vi "KDC101_Goto.vi"(5 "ErrRange(deg)":dbl=0.5, 6 "PositionRef":refnum<vi>, 7 "Position(deg)":dbl, 8 "error in (no error)":errorcluster caption="entrée d'erreur (pas d'erreur)", 9 "MovingRef":refnum<vi>, 10 "StopRef":refnum<vi>, 11 "KCubeDCServoRef":refnum<k24>) -> (0 "error out":errorcluster caption="sortie d'erreur", 1 "In Position":bool, 2 "PositionOut(deg)":dbl, 3 "KCubeDCServoRefOut":refnum<k24>)   [LabVIEW 2019]
doc: "Utilisez ce modèle pour construire un VI à utiliser en tant que sous-VI."
uses:
  C:/Program Files (x86)/National Instruments/LabVIEW 2019/user.lib/ThorKDC101/Kinesis_with_LabVIEW_Examples_LV12 - v3/ThorLabs.MotionControl.KCube.DCServoCLI.dll
  Kinesis_with_LabVIEW_Examples_LV12 - v3/ThorLabs.MotionControl.KCube.DCServoCLI.dll
  C:/Program Files (x86)/National Instruments/LabVIEW 2019/user.lib/ThorKDC101/Kinesis_with_LabVIEW_Examples_LV12 - v3/Thorlabs.MotionControl.GenericMotorCLI.dll
  Kinesis_with_LabVIEW_Examples_LV12 - v3/Thorlabs.MotionControl.GenericMotorCLI.dll
panel:
  in  "Stop":bool
  out "Moving":bool
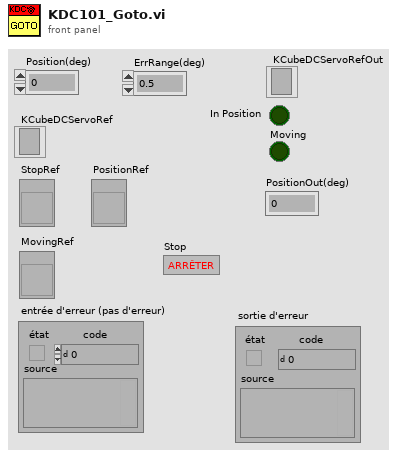
[diagram p1: front panel]
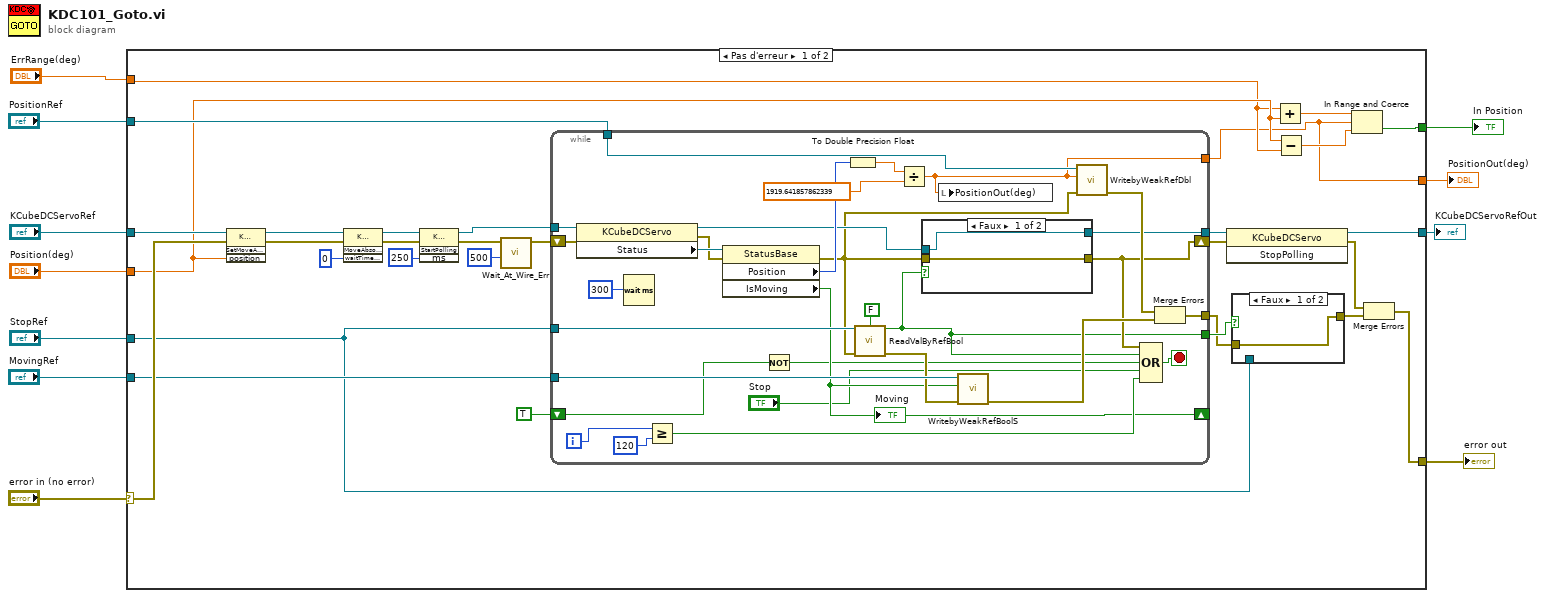
[diagram p0: block diagram]
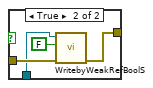
[diagram p2: hidden frame]
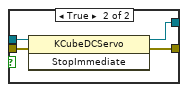
[diagram p3: hidden frame]
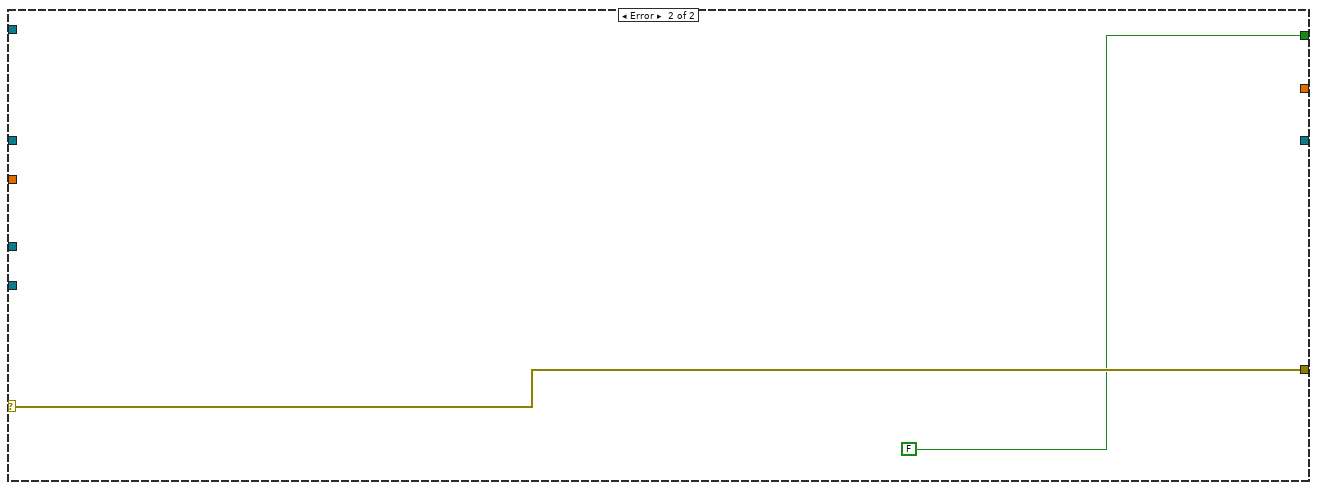
[diagram p4: hidden frame]
diagram:
  n1 = case shown="Pas d'erreur" "error in (no error)" {
    selector: "error in (no error)" -> [w37 w84]
    tunnel: [w33 w84] -> w10
    tunnel: [w17 FALSE] -> w9
    tunnel: "KCubeDCServoRef" -> [w40 _]
    tunnel: "MovingRef" -> [w34 _]
    tunnel: [w31 _] -> w6
    tunnel: "StopRef" -> [w13 _]
    tunnel: "Position(deg)" -> [w21 _]
    tunnel: "PositionRef" -> [w22 _]
    tunnel: "ErrRange(deg)" -> [w20 _]
    tunnel: [w16 _] -> w1
    frame No Error {
      n2 = invoke class="KCubeDCServo" method="SetMoveAbsolutePosition"(reference=w40, error in=w37, "position"=w21) -> (reference out=w27:refnum<k24>, error out=w28:errorcluster)  [unwired: 1 in, 2 out]
      n3 = invoke class="KCubeDCServo" method="MoveAbsolute"(reference=w27, error in=w28, "waitTimeout"=0) -> (reference out=w26:refnum<k24>, error out=w25:errorcluster)  [unwired: 1 in, 2 out]
      n4 = invoke class="KCubeDCServo" method="StartPolling"(reference=w26, error in=w25, "ms"=250) -> (reference out=w35:refnum<k24>, error out=w36:errorcluster)  [unwired: 1 in, 2 out]
      n5 = call <userlib>:"Wait_At_Wire_Err.vi"("Wait (ms)"=u32 500, "error in (no error)"=w36) -> ("error out"=w39:errorcluster)  [unwired: 7 in, 2 out]
      n6 = while {
        tunnel: [w54] -> w32
        tunnel: w35 -> [w75]
        tunnel: w34 -> [w70]
        shift-right: [w56] -> w30
        shift-left: w39 -> [w74]
        tunnel: [w57] -> w14
        tunnel: w13 -> [w69]
        shift-right: [w62] -> _
        shift-left: TRUE ("IsMoving") -> [w51]
        tunnel: w22 -> [w60]
        tunnel: [w48] -> w16
        tunnel: [w47] -> w15
        i -> [w65]
        stop <- w71 stop-if-true
        n7 = property class="KCubeDCServo"(reference=w75, error in=w74) -> (reference out=w55:refnum<k24>, error out=w73:errorcluster, "Status"=w76:refnum<k24>)
        n8 = Wait (ms)(milliseconds to wait=u32 300) -> ()  [unwired: 1 out]
        n9 = Greater Or Equal?(x=w65, y=120 ("x")) -> (x >= y?=w67:bool)
        n10 = property class="StatusBase"(reference=w76, error in=w73) -> (error out=w53:errorcluster, "Position"=w63:i64, "IsMoving"=w62:bool)  [unwired: 1 out]
        "Moving" <- w62
        n11 = Not(x=w51) -> (.not. x?=w50:bool)
        n12 = To Double Precision Float(number=w63) -> (double precision float=w64:dbl)
        n13 = call <userlib>:"ReadValByRefBool.vi"("Control Ref"=w69, "Type In"=FALSE, "error in"=w53) -> ("Valeur"=w47:bool, "error out"=w68:errorcluster)  [unwired: 11 in]
        n14 = Divide(x=w64, y=1919.641857862339) -> (x/y=w48:dbl)
        n15 = case shown="Faux" w47 {
          tunnel: [w77 w82] -> w56
          tunnel: w55 -> [w78 w81]
          tunnel: [w78 w80] -> w54
          tunnel: w53 -> [w77 w79]
          frame False {
          }
          frame True {
            n16 = invoke class="KCubeDCServo" method="StopImmediate"(reference=w81, error in=w79) -> (reference out=w80:refnum<k24>, error out=w82:errorcluster)  [unwired: 1 in, 1 out]
          }
        }
        n17 = local write "PositionOut(deg)"(w48) -> ()
        n18 = call <userlib>:"WritebyWeakRefBoolS.vi"("error in"=w68, "Valeur"=w62, "Control Ref"=w70) -> ("error out"=w58:errorcluster)  [unwired: 8 in]
        n19 = call <userlib>:"WritebyWeakRefDbl.vi"("error in"=w53, "Valeur"=w48, "Control Ref"=w60) -> ("error out"=w59:errorcluster)  [unwired: 8 in]
        n20 = Compound Arithmetic op=OR ("Opérateur arithmétique")(w56, w47, w50, "Stop", w67) -> (w71:bool)
        n21 = Merge Errors(w59, w58) -> (w57:errorcluster)
      }
      n22 = invoke class="KCubeDCServo" method="StopPolling"(reference=w32, error in=w30) -> (reference out=w31:refnum<k24>, error out=w29:errorcluster)  [unwired: 1 in, 1 out]
      n23 = case shown="Faux" w15 {
        tunnel: w14 -> [w42 w46]
        tunnel: [w42 w43] -> w12
        tunnel: w13 -> [_ w44]
        frame False {
        }
        frame True {
          n24 = call <userlib>:"WritebyWeakRefBoolS.vi"("error in"=w46, "Valeur"=FALSE, "Control Ref"=w44) -> ("error out"=w43:errorcluster)  [unwired: 8 in]
        }
      }
      n25 = Add(x=w20, y=w21) -> (x+y=w19:dbl)
      n26 = Subtract(x=w21, y=w20) -> (x-y=w18:dbl)
      n27 = In Range and Coerce(upper limit=w19, x=w16, lower limit=w18) -> (In Range?=w17:bool)  [unwired: 1 out]
      n28 = Merge Errors(w29, w12) -> (w33:errorcluster)
    }
    frame Error {
    }
  }
  "error out" <- w10
  "In Position" <- w9
  "KCubeDCServoRefOut" <- w6
  "PositionOut(deg)" <- w1
